vi "Configure Limit.vi"(6 "Lower Limit Value (0 Hz)":dbl, 7 "Upper Limit Value (0 Hz)":dbl, 8 "error in (no error)":errorcluster, 9 "Enable Calculate1 (T: Enable)":bool=TRUE, 10 "Enable Limit Test (T: Enable)":bool=TRUE, 11 "VISA resource name":refnum<visa-resource-name>) -> (0 "error out":errorcluster, 3 "VISA resource name out":refnum<visa-resource-name>)   [LabVIEW 2021, in "Agilent 532XX Series.lvlib"]
doc: "Configures the parameters required for post acquisition Limit testing."
uses:
  <instrlib>/Agilent 532XX Series/Agilent 532XX Series.lvlib
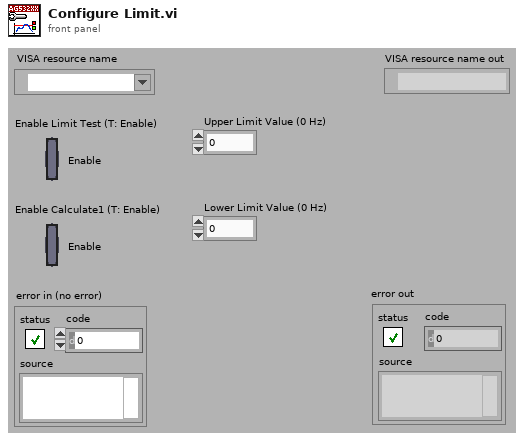
[diagram p1: front panel]
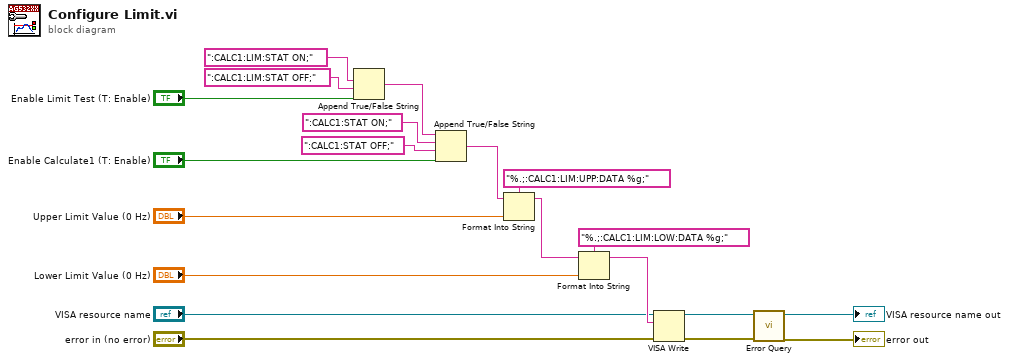
[diagram p0: block diagram]
diagram:
  n1 = Append True/False String(1:"Enable Limit Test (T: Enable)", 2:":CALC1:LIM:STAT OFF;", 3:":CALC1:LIM:STAT ON;") -> (0:w17:string)  [unwired: 1 out]
  n2 = Append True/False String(1:"Enable Calculate1 (T: Enable)", 2:":CALC1:STAT OFF;", 3:":CALC1:STAT ON;", 4:w17) -> (0:w13:string)
  n3 = Format Into String(format string="%.;:CALC1:LIM:UPP:DATA %g;", initial string=w13, "Upper Limit Value (0 Hz)") -> (resulting string=w10:string)  [unwired: 1 in, 1 out]
  n4 = Format Into String(format string="%.;:CALC1:LIM:LOW:DATA %g;", initial string=w10, "Lower Limit Value (0 Hz)") -> (resulting string=w7:string)  [unwired: 1 in, 1 out]
  n5 = VISA Write(VISA resource name="VISA resource name", write buffer=w7, error in (no error)="error in (no error)") -> (VISA resource name out=w4:refnum<visa-resource-name>, error out=w3:errorcluster)  [unwired: 1 out]
  n6 = call <instrlib>:"Error Query.vi"("error in (no error)"=w3, "VISA resource name"=w4) -> ("error out"=→"error out":errorcluster, "VISA resource name out"=→"VISA resource name out":refnum<visa-resource-name>)  [unwired: 8 out]
